vi "NewBallLifetime.vi"(10 "last balls":T1[](array[typedef]), 11 "current ball":T1[](array[typedef])) -> (3 "balls out":T1[](array[typedef]))   [LabVIEW 2023]
uses:
  Old vision/Controls/SSL Detection Ball.ctl
  <vilib>/Analysis/Matrix/Datatypes/RealMatrix.ctl
  <vilib>/Analysis/Matrix/NI_Matrix.lvlib
panel:
  in  "Life Time":dbl=2.0
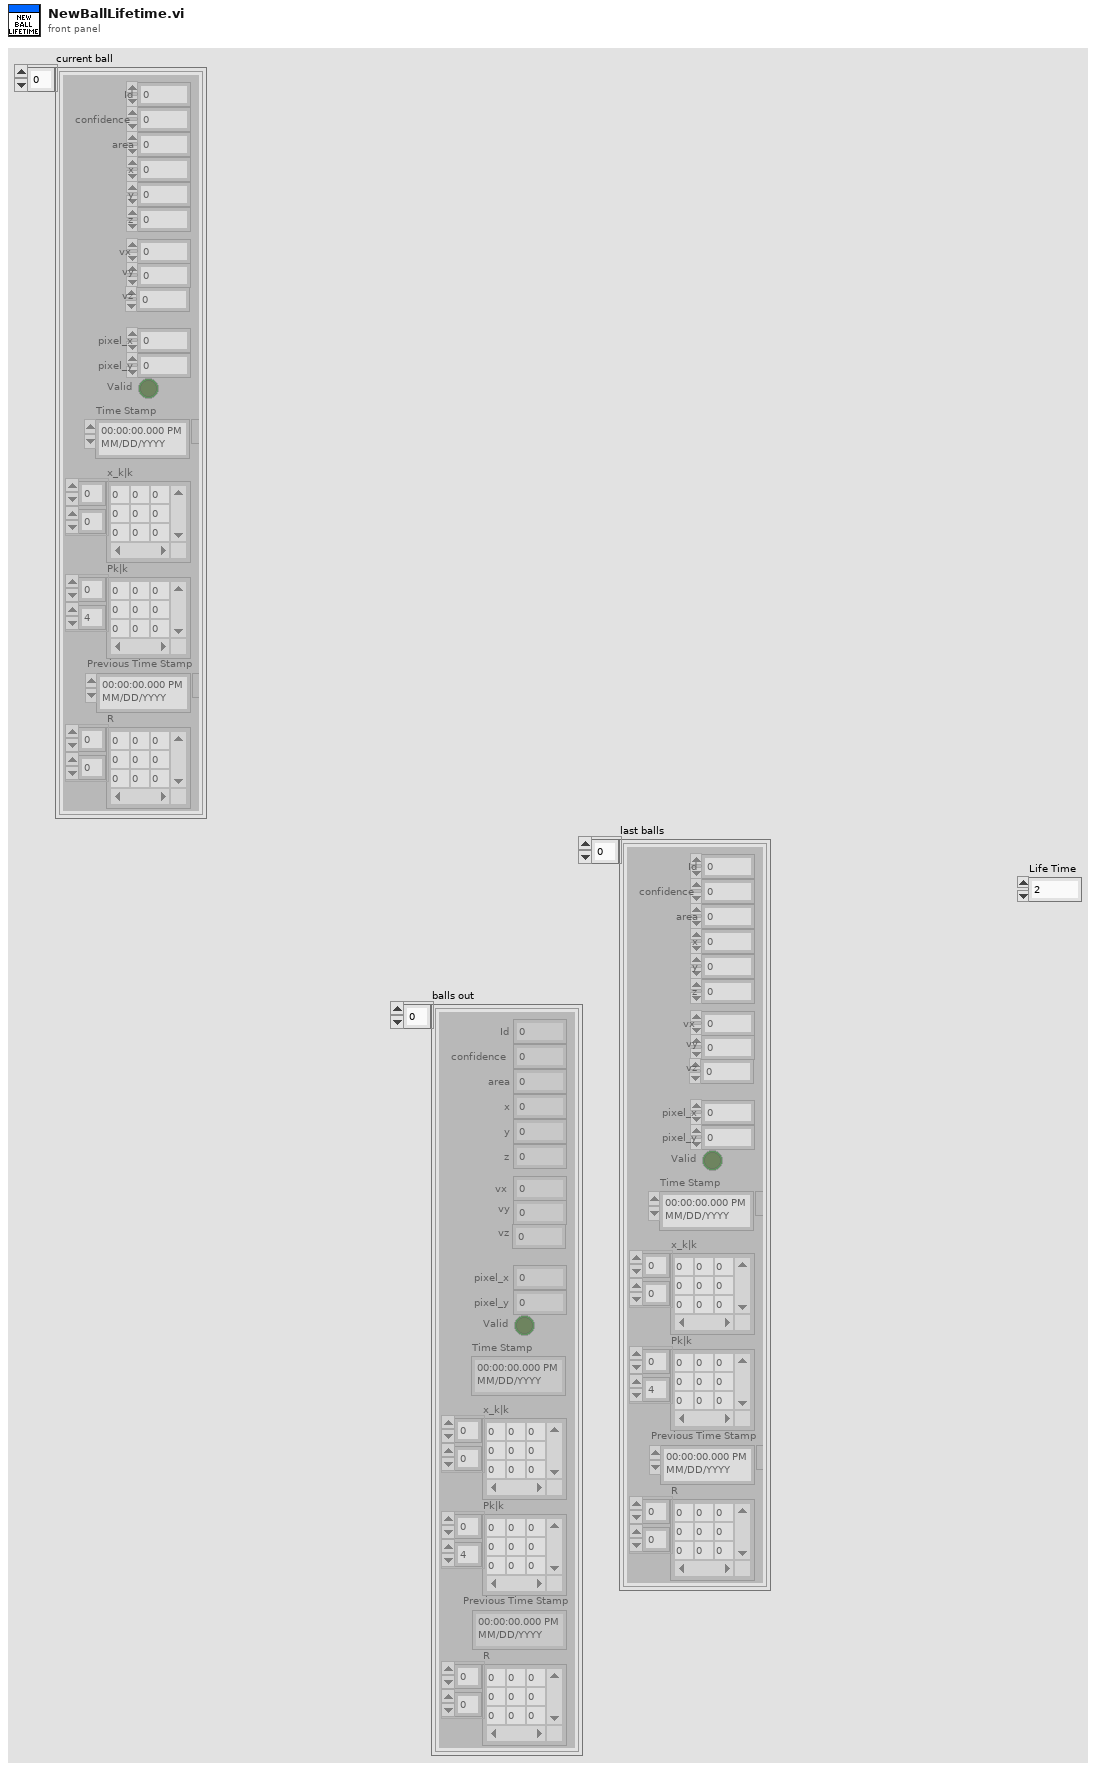
[diagram p1: front panel]
types:
  T1 = typedef "SSL Detection Ball.ctl" = cluster{"x":sgl, "area":u32, "confidence":sgl, "y":sgl, "z":sgl, "pixel_x":sgl, "pixel_y":sgl, "Valid":bool, "Time Stamp":timestamp, "x_k|k":T2, "Pk|k":T2, "Id":u32, "Previous Time Stamp":timestamp, "R":T2, " vx":sgl, "vy":dbl, "vz":dbl}
  T2 = typedef "NI_Matrix.lvlib/RealMatrix.ctl" = dbl[][]
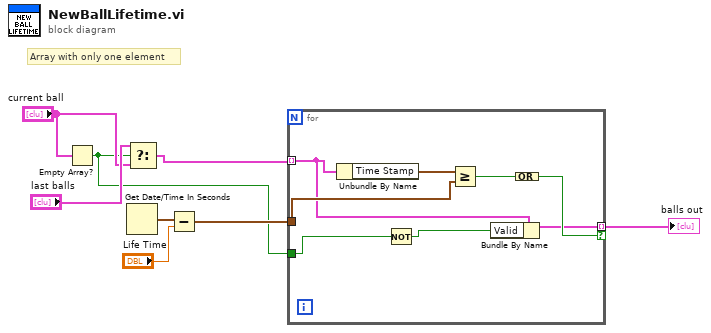
[diagram p0: block diagram]
diagram:
  # "Array with only one element"
  n1 = Empty Array?(array="current ball") -> (empty?=w2:bool)
  n2 = Get Date/Time In Seconds() -> (seconds since 1Jan1904=w8:timestamp)
  n3 = Select(t="last balls", s=w2, f="current ball") -> (s? t:f=w3:T1[])
  n4 = Subtract(x=w8, y="Life Time") -> (x-y=w6:timestamp)
  n5 = for {
    tunnel: w3 -> [w11] mode=indexing
    tunnel: [w12] -> w1 mode=indexing if=w16
    tunnel: w6 -> [w13]
    tunnel: w2 -> [w10]
    n6 = Unbundle By Name(w11) -> ("Time Stamp"=w15:timestamp)
    n7 = Not(x=w10) -> (.not. x?=w9:bool)
    n8 = Greater Or Equal?(x=w15, y=w13) -> (x >= y?=w14:bool)
    n9 = Bundle By Name(cluster=w11, "Valid"=w9) -> (w12:T1)
    n10 = Compound Arithmetic op=OR(w14) -> (w16:bool)
  }
  "balls out" <- w1
